vi "Bode_Magnitude_Plot.vi"() -> ()   [LabVIEW 2015]
uses:
  <vilib>/Analysis/NI_AALPro.lvlib
panel:
  out "XY Graph":cluster{i32[], dbl[]}(graph)
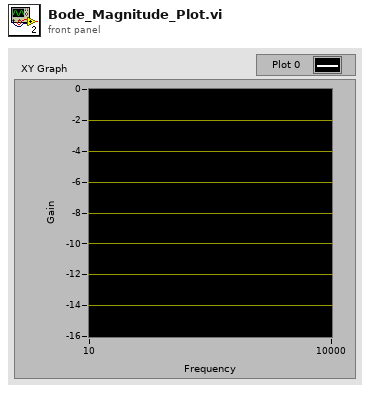
[diagram p1: front panel]
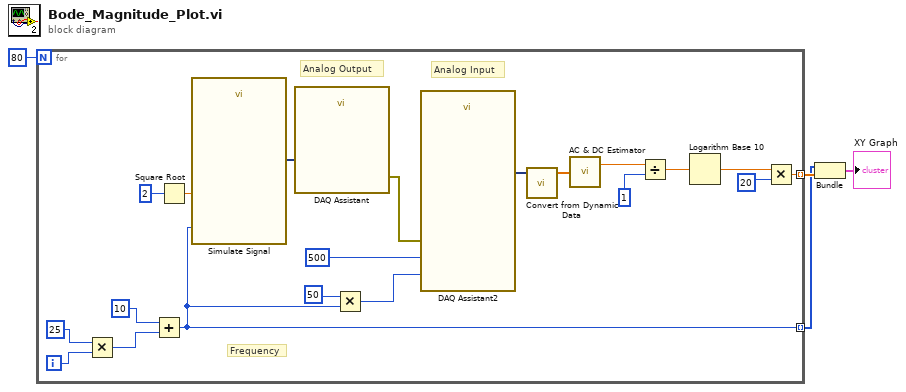
[diagram p0: block diagram]
diagram:
  n1 = for {
    N: 80 -> [_]
    tunnel: [w6] -> w2 mode=indexing
    tunnel: [w5] -> w1 mode=indexing
    i -> [w24]
    # "Frequency"
    # "Analog Input"
    # "Analog Output"
    n2 = Multiply(x=25, y=w24) -> (x*y=w22:i32)
    n3 = Add(x=10, y=w22) -> (x+y=w5:i32)
    n4 = Square Root(x=2) -> (sqrt(x)=w19:dbl)
    n5 = call "Simulate Signal"("Frequency"=w5, "Amplitude"=w19) -> ("Sine"=w18:dynamicdata)  [unwired: 12 in, 1 out]
    n6 = call "DAQ Assistant"("data"=w18) -> ("error out"=w17:errorcluster)  [unwired: 16 in, 2 out]
    n7 = Multiply(x=50, y=w5) -> (x*y=w15:i32)
    n8 = call "DAQ Assistant2"("rate"=w15, "number of samples"=500, "error in"=w17) -> ("data"=w13:dynamicdata)  [unwired: 14 in, 2 out]
    n9 = call "Convert from Dynamic Data"("Dynamic Data Type"=w13) -> ("Array"=w12:dbl[])  [unwired: 3 in]
    n10 = call <vilib>:"AC & DC Estimator.vi"("Signal (V)"=w12) -> ("AC estimate (Vrms)"=w8:dbl)  [unwired: 1 out]
    n11 = Divide(x=w8, y=1) -> (x/y=w11:dbl)
    n12 = Logarithm Base 10(1:w11) -> (0:w10:dbl)
    n13 = Multiply(x=w10, y=20) -> (x*y=w6:dbl)
  }
  n14 = Bundle(w1, w2) -> (→"XY Graph":cluster{i32[], dbl[]})  [unwired: 1 in]
